vi "Obtain Set-Point Driver Notifier.vi"() -> (0 "Set-Point Driver Notifier":refnum<notifier>)   [LabVIEW 2013]
uses:
  Set-Point Driver Messages.ctl
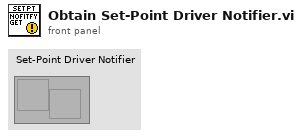
[diagram p1: front panel]
types:
  T1 = typedef "Set-Point Driver Messages.ctl" = enum16{"Begin Enforcement", "Cease Enforcement"}
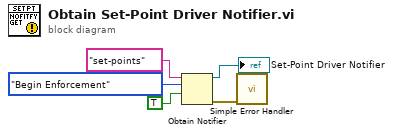
[diagram p0: block diagram]
diagram:
  n1 = Obtain Notifier(name (unnamed)="set-points", notification data type=Set-Point_Driver_Messages."Begin Enforcement", create if not found? (T)=TRUE) -> (notifier out=→"Set-Point Driver Notifier":refnum<notifier>, error out=w2:errorcluster)  [unwired: 1 in, 1 out]
  n2 = call <vilib>:"Simple Error Handler.vi"("error in (no error)"=w2) -> ()  [unwired: 4 in, 5 out]
